vi "Read Handle.vi"(8 "Error In":errorcluster, 11 "Identity In":refnum<class "Agent Identity.lvclass">) -> (0 "Error Out":errorcluster, 2 "Handle":u64, 3 "Identity Out":refnum<class "Agent Identity.lvclass">)   [LabVIEW 2018, in "Toolkit.lvlib" / "Agent Identity.lvclass"]
uses:
  Agent Identity.lvclass
  Agent Identity.lvclass/Agent Identity.ctl
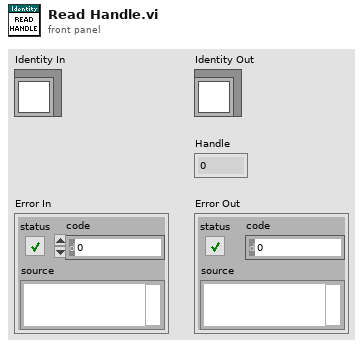
[diagram p1: front panel]
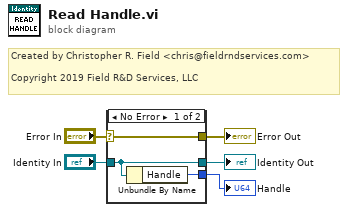
[diagram p0: block diagram]
diagram:
  # "Created by Christopher R. Field <chris@fieldrndservices.com>\n\nCopyright 2019 Field R&D Services, LLC"
  n1 = case shown="No Error" "Error In" {
    selector: "Error In" -> [w7 w10]
    tunnel: "Identity In" -> [w8 w9]
    tunnel: [w8 w9] -> w1
    tunnel: [w7 w10] -> w4
    tunnel: [w6 _] -> w3
    frame No Error {
      n2 = Unbundle By Name(w8) -> ("Handle"=w6:u64)
    }
    frame Error {
    }
  }
  "Error Out" <- w4
  "Handle" <- w3
  "Identity Out" <- w1
